vi "Smite.vi"(8 "Error In":errorcluster) -> (0 "Error Out":errorcluster)   [LabVIEW 2018, in "Tests.lvlib" / "Toolkit.lvlib" / "Integration.lvlib"]
uses:
  Integration.lvlib
  <vilib>/addons/_JKI Toolkits/Caraya/classes/Test/Test.lvclass
  <vilib>/addons/_JKI Toolkits/Caraya/classes/Assert/Assert.lvclass
  src/Toolkit/Toolkit.lvlib
  Tests.lvlib
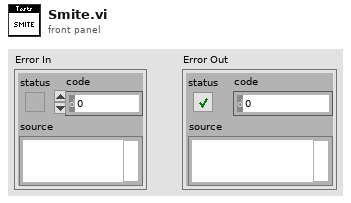
[diagram p1: front panel]
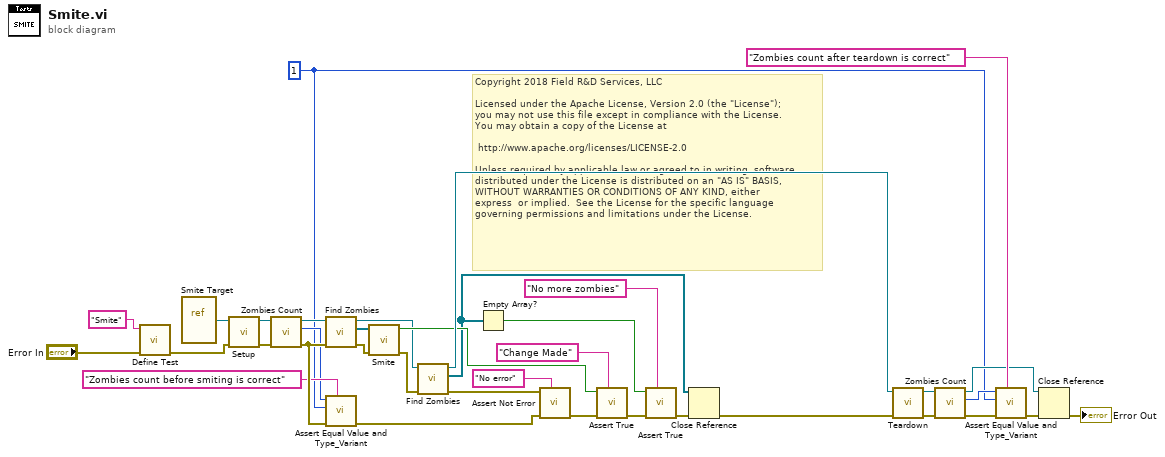
[diagram p0: block diagram]
diagram:
  w1 = 1 ("Zombies Count")
  # "Copyright 2018 Field R&D Services, LLC\n\nLicensed under the Apache License, Version 2.0 (the \"License\");\nyou may not use this file except in compliance with the License.\nYou may obtain a copy of the License at\n\n\thttp://www.apache.org/licenses/LICENSE-2.0\n\nUnless required by applicable law or agreed to in writing, software\ndistributed under the License is distributed on an \"AS IS\" BASIS,\nWITHOUT WARRANTIES OR CONDITIONS OF ANY KIND, either \nexpress  or implied.  See the License for the specific language \ngoverning permissions and limitations under the License."
  n1 = call <vilib>:"Define Test.vi"("error in (no error)"="Error In", "Label (VI Title)"="Smite") -> ("error out"=w17:errorcluster)  [unwired: 9 in]
  n2 = vi-ref "Smite Target.vi"() -> (w20:refnum<vi>)
  n3 = call "Setup.vi"("Error In"=w17, "VI In"=w20) -> ("Error Out"=w7:errorcluster, "VI Out"=w8:refnum<vi>)  [unwired: 8 in]
  n4 = call "Zombies Count.vi"("Error In"=w7, "Test Target In"=w8) -> ("Error Out"=w6:errorcluster, "Zombies Count"=w2:i32, "Test Target Out"=w3:refnum<vi>)  [unwired: 7 in]
  n5 = call "Find Zombies.vi"("Error In"=w6, "VI In"=w3) -> ("Error Out"=w23:errorcluster, "Graves"=w21:refnum<vi>[], "VI Out"=w22:refnum<vi>)  [unwired: 7 in]
  n6 = call <vilib>:"Assert Equal Value and Type_Variant.vi"("Label"="Zombies count before smiting is correct", "error in (no error)"=w6, "Y"=w1, "X"=w2) -> ("error out"=w5:errorcluster)  [unwired: 7 in]
  n7 = call "Smite.vi"("Error In"=w23, "Graves"=w21) -> ("Error Out"=w36:errorcluster, "Change Made?"=w25:bool)  [unwired: 8 in]
  n8 = call "Find Zombies.vi"("Error In"=w36, "VI In"=w22) -> ("Error Out"=w31:errorcluster, "Graves"=w18:refnum<vi>[], "VI Out"=w28:refnum<vi>)  [unwired: 7 in]
  n9 = Empty Array?(array=w18) -> (empty?=w19:bool)
  n10 = call <vilib>:"Assert Not Error.vi"("Label"="No error", "error in (no error)"=w5, "Not Error?"=w31) -> ("error out"=w33:errorcluster)  [unwired: 8 in]
  n11 = call <vilib>:"Assert True.vi"("Label"="Change Made", "error in (no error)"=w33, "True?"=w25) -> ("error out"=w26:errorcluster)  [unwired: 8 in]
  n12 = call <vilib>:"Assert True.vi"("Label"="No more zombies", "error in (no error)"=w26, "True?"=w19) -> ("error out"=w29:errorcluster)  [unwired: 8 in]
  n13 = Close Reference(reference=w18, error in (no error)=w29) -> (error out=w16:errorcluster)
  n14 = call "Teardown.vi"("Error In"=w16, "VI In"=w28) -> ("Error Out"=w15:errorcluster, "VI Out"=w14:refnum<vi>)  [unwired: 8 in]
  n15 = call "Zombies Count.vi"("Error In"=w15, "Test Target In"=w14) -> ("Error Out"=w13:errorcluster, "Zombies Count"=w12:i32, "Test Target Out"=w9:refnum<vi>)  [unwired: 7 in]
  n16 = call <vilib>:"Assert Equal Value and Type_Variant.vi"("Label"="Zombies count after teardown is correct", "error in (no error)"=w13, "Y"=w1, "X"=w12) -> ("error out"=w10:errorcluster)  [unwired: 7 in]
  n17 = Close Reference(reference=w9, error in (no error)=w10) -> (error out=→"Error Out":errorcluster)
